vi "16进制至正常显示.vi"(11 "字符串_16进制":string) -> (2 "字符串_正常":string)   [LabVIEW 2010]
panel:
  # "用于串口读数据"
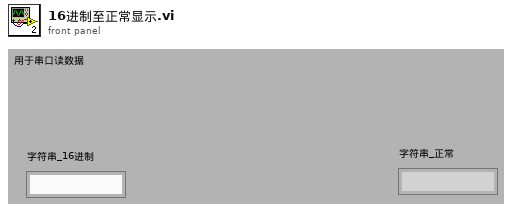
[diagram p1: front panel]
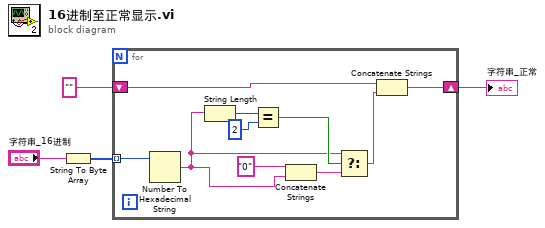
[diagram p0: block diagram]
diagram:
  n1 = String To Byte Array(string="字符串_16进制") -> (unsigned byte array=w3:u8[])
  n2 = for {
    tunnel: w3 -> [w14] mode=indexing
    shift-right: [w6] -> w1
    shift-left: "" -> [w7]
    n3 = Number To Hexadecimal String(2:w14) -> (0:w8:string)  [unwired: 1 in]
    n4 = String Length(string=w8) -> (length=w13:i32)
    n5 = Equal?(x=w13, y=2) -> (x = y?=w10:bool)
    n6 = Concatenate Strings("0", w8) -> (w11:string)
    n7 = Select(t=w8, s=w10, f=w11) -> (s? t:f=w5:string)
    n8 = Concatenate Strings(w7, w5) -> (w6:string)
  }
  "字符串_正常" <- w1
